vi "Test Bench v18 - TDMS.vi"(5 "Folder to save file to":path=path "C:/Users/LAV-UFSC-2023/Documents/LAV-TCC/Dados-Experimentos/Dados-Bancada-LABVIEW", 6 "Signal Output\nControl":enum32{"White Noise", "Harmonic"}(tab), 7 "stop":bool, 8 "Enable Display":bool=TRUE, 9 "Accel. 2":bool, 10 "Output":bool=TRUE) -> (0 "New file path":path, 2 "Accel. 1 Raw":dbl[](graph), 3 "Output Signal":dynamicdata(graph))   [LabVIEW 2022 SP3]
uses:
  WhiteNoise.ctl
  <vilib>/Utility/error.llb/DialogType.ctl
  <vilib>/Platform/TimedLoop/XDataNode/timing_clust.ctl
  <vilib>/Platform/TimedLoop/XDataNode/nitl_modes.ctl
  <vilib>/Platform/TimedLoop/XDataNode/wakeup.ctl
  <vilib>/DAQmx/write.llb/DAQmx Write (Analog 2D DBL NChan NSamp).vi
  <vilib>/DAQmx/read.llb/DAQmx Read (Analog 1D DBL 1Chan NSamp).vi
  <vilib>/DAQmx/create/channels.llb/DAQmx Create Channel (AI-Acceleration-Accelerometer).vi
  <vilib>/DAQmx/create/channels.llb/DAQmx Create Channel (AO-Voltage-Basic).vi
  <vilib>/DAQmx/configure/timing.llb/DAQmx Timing (Sample Clock).vi
  <vilib>/DAQmx/miscellaneous.llb/DAQmx Fill In Error Info.vi
  <vilib>/platform/TimedLoop/XDataNode/XDataNode.xnode
  <vilib>/measure/NI_MABase.lvlib
  <vilib>/Platform/TimedLoop/XDataNode/XDNodeRunTimeDep.lvlib
  <resource>/objmgr/daqmx.rc
panel:
  in  "Sample Rate":dbl=41200.0
  in  "samples per channel":i32=41200
  out "Frame 2 Duration":i64
  out "Frame 1 Duration":i64
  in  "White Noise\nParameters":T2={"Seed"=0.0, "Standard Deviation"=2.0, "Reset"=FALSE, "Iterator"=1.0, "Seed"=-1, "Lower Cut-Off"=5.0, "Upper Cut-Off"=350.0} {"Upper Cut-Off" min=5.0 max=350.0 step=10.0; "Lower Cut-Off" min=5.0 max=350.0 step=10.0; "Standard Deviation" min=0.001 max=3.0 step=0.05 format="%0.2p"}
  in  "Hamonic\nParameters":T3={"Waveform Type"=0, "Frequency"=10.0, "Amplitude"=0.25} {"Frequency" min=5.0 max=350.0 step=10.0 format="%0.2p"; "Waveform Type" items=["Sine Wave", "Triangle Wave", "Square Wave", "Sawtooth Wave"]; "Amplitude" min=0.001 max=0.3 step=0.05 format="%0.2p"}
  # "Filter"
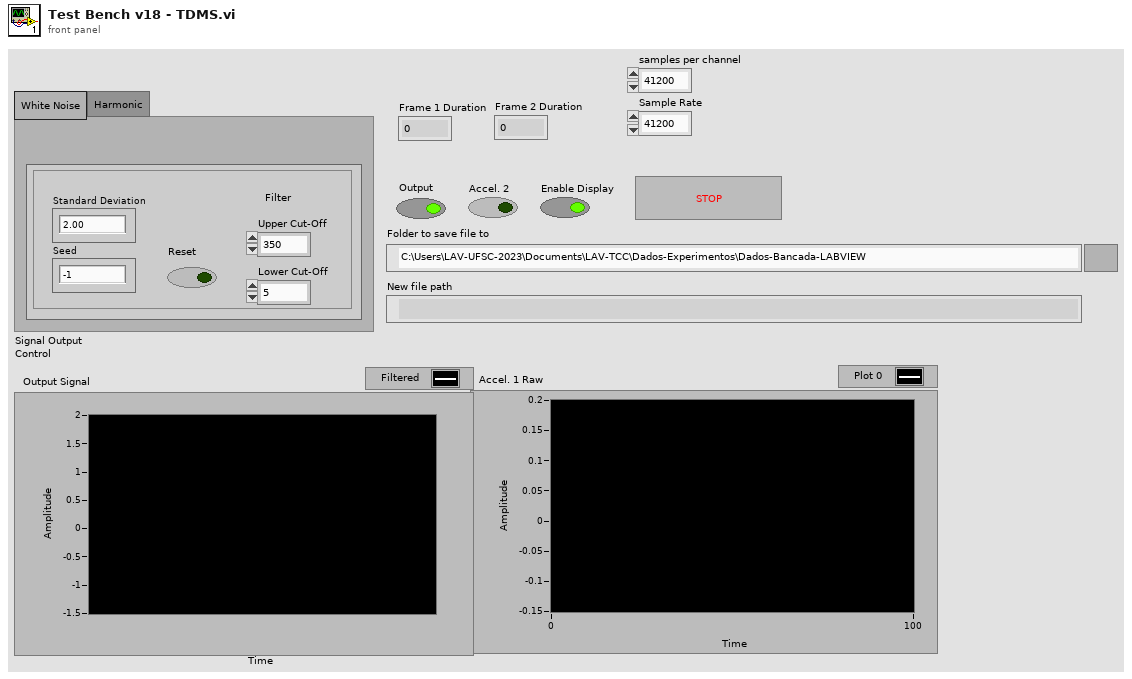
[diagram p1: front panel]
types:
  T1 = typedef "WhiteNoise.ctl" = dbl
  T2 = cluster{"Seed":T1, "Standard Deviation":dbl, "Reset":bool, "Iterator":dbl, "Seed":i8, "Lower Cut-Off":dbl, "Upper Cut-Off":dbl}
  T3 = cluster{"Waveform Type":u16, "Frequency":dbl, "Amplitude":dbl}
  T4 = typedef "DialogType.ctl" = u16
  T5 = enum16{"open", "open or create", "create or replace", "create", "open (read-only)"}
  T6 = typedef "XDNodeRunTimeDep.lvlib/timing_clust.ctl" = cluster{"Expected End [f-1]":u64, "Actual End [f-1]":u64, "Finished Late? [f-1]":bool, "Expected End [i-1]":u64, "Actual End [i-1]":u64, "Finished Late? [i-1]":bool, "Expected Start [i]":u64, "Actual Start [i]":u64, "Expected Start [f]":u64, "Actual Start [f]":u64, "Source Name":string, "Structure Name":string, "Period":i64, "Deadline":i64, "Offset":i64, "Start":i64, "Priority":i32, "Timeout":i32, "Mode":T7, "Wakeup Reason":T8, "Error":errorcluster, "Source Type":string, "Secondary Source Type":string, "Global End Time":u64, "Global Start Time":u64, "Frame Duration":u64, "Iteration Duration":u64, "Assigned CPU":i32, "I/O Scan Engine Mode":u32}
  T7 = typedef "XDNodeRunTimeDep.lvlib/nitl_modes.ctl" = enum32{"No Change", "Process missed periods, maintain original phase", "Discard missed periods, maintain original phase", "Process missed periods, ignore original phase", "Discard missed periods, ignore original phase"}
  T8 = typedef "XDNodeRunTimeDep.lvlib/wakeup.ctl" = enum32{"Normal", "Aborted", "Asynchronous wakeup", "Timing source error", "Timed loop error", "Timeout"}
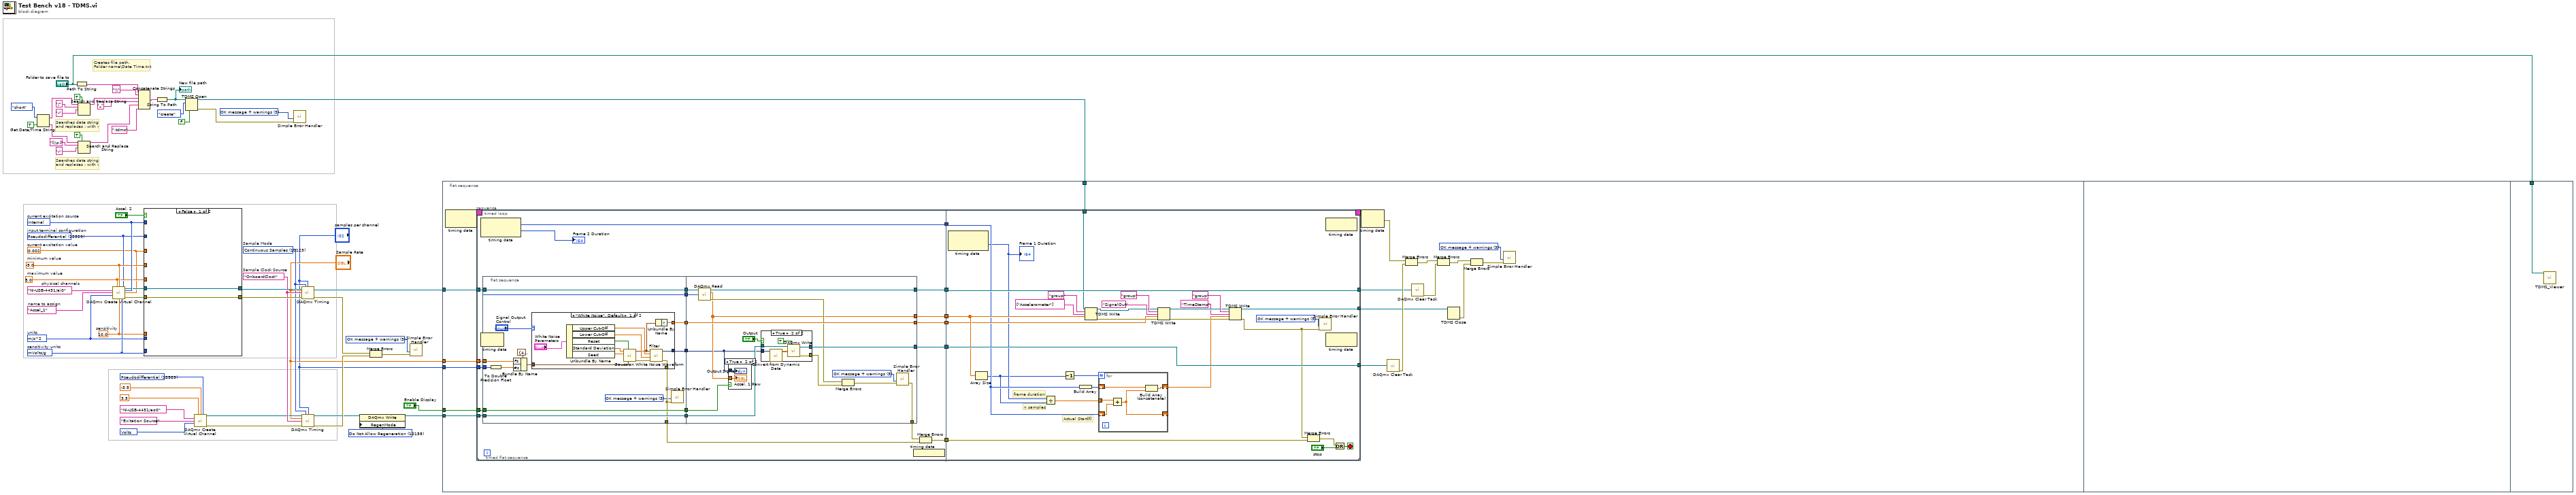
[diagram p0: block diagram]
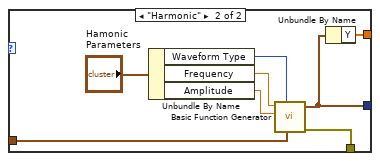
[diagram p2: hidden frame]
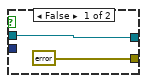
[diagram p4: hidden frame]
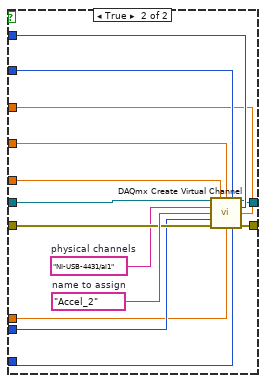
[diagram p5: hidden frame]
diagram:
  w1 = 10158 items=["Allow Regeneration"=10097, "Do Not Allow Regeneration"=10158] ("RegenMode")
  w13 = T4 3 items=["no dialog", "OK message", "continue or stop message", "OK message + warnings", "continue/stop + warnings"] ("type of dialog (OK msg:1)")
  w15 = T4 3 items=["no dialog", "OK message", "continue or stop message", "OK message + warnings", "continue/stop + warnings"] ("type of dialog (OK msg:1)")
  w47 = 12529 items=["Default"=-1, "RSE"=10083, "Differential"=10106, "Pseudodifferential"=12529] ("output terminal configuration")
  w45 = 10348 items=["Volts"=10348, "From Custom Scale"=10065] ("units")
  w51 = 12509 items=["mVolts/g"=12509, "Volts/g"=12510]  # sensitivity units
  w42 = 10.0  # sensitivity
  w50 = 0.002  # current excitation value
  w58 = 10200 items=["Internal"=10200, "External"=10167, "None"=10230]  # current excitation source
  w52 = tag "NI-USB-4431/ai0"  # physical channels
  w39 = tag "OnboardClock"  # Sample Clock Source
  w38 = 10123 items=["Finite Samples"=10178, "Continuous Samples"=10123, "Hardware Timed Single Point"=12522]  # Sample Mode
  w54 = 12529 items=["default"=-1, "RSE"=10083, "NRSE"=10078, "Differential"=10106, "Pseudodifferential"=12529]  # input terminal configuration
  w57 = -5.0  # minimum value
  w56 = 5.0  # maximum value
  w60 = "Accel_1"  # name to assign
  w55 = 12470 items=["g"=10186, "m/s^2"=12470, "in/s^2"=12471, "From Custom Scale"=10065]  # units
  # "Searches date string\nand replaces : with -"
  # "Searches date string\nand replaces : with -"
  # "Creates file path.\nFolder name\\Date Time.txt"
  n1 = Get Date/Time String(date format (0)=enum16{"short", "long", "abbreviated"}."short", want seconds? (F)=TRUE) -> (date string=w18:string, time string=w31:string)  [unwired: 1 in]
  n2 = Path To String(path="Folder to save file to") -> (string=w26:string)
  n3 = Search and Replace String(replace all?=TRUE ("replace all? (F)"), input string=w18, search string="/" ("replace string (\"\")"), replace string="-" ("replace string (\"\")")) -> (result string=w17:string)  [unwired: 4 in, 3 out]
  n4 = Search and Replace String(replace all?=TRUE ("replace all? (F)"), input string=w31, search string="[\\s:]" ("replace string (\"\")"), replace string="-" ("replace string (\"\")")) -> (result string=w24:string)  [unwired: 4 in, 3 out]
  n5 = call-poly <vilib>:"DAQmx Create Virtual Channel.vi"("maximum value"=w56, "minimum value"=w57, "input terminal configuration"=w54, "physical channels"=w52, "current excitation source"=w58, "name to assign"=w60, "current excitation value"=w50, "units"=w55, "sensitivity"=w42, "sensitivity units"=w51) -> ("task out"=w53:refnum<k21>, "error out"=w59:errorcluster)  [unwired: 4 in]
  n6 = Concatenate Strings(w26, "\\" ("string"), w17, "_" ("string"), w24, ".tdms" ("string")) -> (w22:string)
  n7 = case shown="False" "Accel. 2" {
    tunnel: w59 -> [w62 w75]
    tunnel: w58 -> [_ w74]
    tunnel: w57 -> [_ w73]
    tunnel: w56 -> [_ w72]
    tunnel: w55 -> [_ w71]
    tunnel: w54 -> [_ w70]
    tunnel: w53 -> [w61 w69]
    tunnel: w51 -> [_ w67]
    tunnel: w50 -> [_ w66]
    tunnel: w42 -> [_ w65]
    tunnel: [w62 w64] -> w41
    tunnel: [w61 w63] -> w40
    frame False {
    }
    frame True {
      w68 = tag "NI-USB-4431/ai1"  # physical channels
      w76 = "Accel_2"  # name to assign
      n8 = call-poly <vilib>:"DAQmx Create Virtual Channel.vi"("task in"=w69, "maximum value"=w72, "minimum value"=w73, "input terminal configuration"=w70, "physical channels"=w68, "current excitation source"=w74, "name to assign"=w76, "current excitation value"=w66, "units"=w71, "error in"=w75, "sensitivity"=w65, "sensitivity units"=w67) -> ("task out"=w63:refnum<k21>, "error out"=w64:errorcluster)  [unwired: 2 in]
    }
  }
  n9 = String To Path(string=w22) -> (path=w8:path)
  "New file path" <- w8
  n10 = TDMS Open(6:FALSE ("enable asynchronous? (T)"), 10:T5."create" ("operation (0:open)"), 11:w8) -> (0:w4:errorcluster, 3:w5:refnum<k34>)  [unwired: 4 in]
  n11 = call-poly <vilib>:"DAQmx Create Virtual Channel.vi"("maximum value"=3.5, "minimum value"=-3.5, "output terminal configuration"=w47, "physical channels"=tag "NI-USB-4431/ao0", "name to assign"="Exitation Source", "units"=w45) -> ("task out"=w36:refnum<k21>, "error out"=w37:errorcluster)  [unwired: 8 in]
  n12 = call <vilib>:"Simple Error Handler.vi"("type of dialog (OK msg:1)"=w15, "error in (no error)"=w4) -> ()  [unwired: 3 in, 5 out]
  n13 = call-poly <vilib>:"DAQmx Timing.vi"("task/channels in"=w40, "sample mode"=w38, "samples per channel"="samples per channel", "rate"="Sample Rate", "source"=w39, "error in"=w41) -> ("task out"=w12:refnum<k21>, "error out"=w44:errorcluster)  [unwired: 8 in]
  n14 = call-poly <vilib>:"DAQmx Timing.vi"("task/channels in"=w36, "sample mode"=w38, "samples per channel"="samples per channel", "rate"="Sample Rate", "source"=w39, "error in"=w37) -> ("task out"=w3:refnum<k21>, "error out"=w35:errorcluster)  [unwired: 8 in]
  n15 = property class="DAQmx Write"(reference=w3, "RegenMode"=w1) -> (reference out=w2:refnum<k21>)  [unwired: 1 in, 1 out]
  n16 = Merge Errors(w44, w35) -> (w11:errorcluster)
  n17 = call <vilib>:"Simple Error Handler.vi"("type of dialog (OK msg:1)"=w13, "error in (no error)"=w11) -> ()  [unwired: 3 in, 5 out]
  n18 = flat-sequence {
    tunnel: w2 -> [w92]
    tunnel: w12 -> [w90]
    tunnel: w5 -> [w82]
    tunnel: "Enable Display" -> [w89]
    tunnel: "Sample Rate" -> [w81]
    tunnel: "samples per channel" -> [w80]
    tunnel: "Folder to save file to" -> [w243]
    frame #0 {
      w93 = T4 3 items=["no dialog", "OK message", "continue or stop message", "OK message + warnings", "continue/stop + warnings"] ("type of dialog (OK msg:1)")
      n19 = node-c288() -> (w95:T6)  [unwired: 1 in]
      n20 = timed-loop {
        tunnel: w92 -> [w104]
        tunnel: [w103] -> w91
        tunnel: w90 -> [w102]
        tunnel: [w98] -> w87
        tunnel: [w96] -> w79
        tunnel: w89 -> [w101]
        tunnel: w80 -> [w100]
        timing: w95 -> [_]
        timing-out: [_] -> w94
        tunnel: w82 -> [w99]
        tunnel: w81 -> [w97]
        stop <- w225 stop-if-true
        n21 = timed-sequence {
          timing: _ -> [_]
          timing-out: _ -> [_]
          tunnel: w104 -> [w119]
          tunnel: [w118] -> w103
          tunnel: w102 -> [w117]
          tunnel: w101 -> [w116]
          tunnel: w100 -> [w115]
          tunnel: w99 -> [w111]
          tunnel: [w110] -> w98
          tunnel: w97 -> [w107]
          tunnel: [w106] -> w96
          n22 = timed-flat-sequence {
            tunnel: w119 -> [w133]
            tunnel: w117 -> [w132]
            tunnel: w116 -> [w129]
            tunnel: w115 -> [w128]
            tunnel: [w131] -> w114
            tunnel: [w130] -> w113
            tunnel: [w125] -> w112
            tunnel: [w124] -> w109
            tunnel: [w123] -> w108
            tunnel: w107 -> [w122]
            tunnel: [w121] -> w105
            tunnel: [w229] -> w118
            tunnel: w114 -> [w229]
            tunnel: w113 -> [w223]
            tunnel: w112 -> [w226]
            tunnel: w111 -> [w212]
            tunnel: [w223] -> w110
            tunnel: w109 -> [w221]
            tunnel: w108 -> [w213]
            tunnel: [w217] -> w106
            tunnel: w105 -> [w206]
            frame #0 {
              n23 = node-c288() -> (w121:i64, →"Frame 2 Duration":i64)  [unwired: 1 in]
              n24 = flat-sequence {
                tunnel: [w153] -> w139
                tunnel: [w149] -> w138
                tunnel: [w152] -> w137
                tunnel: [w150] -> w136
                tunnel: [w151] -> w135
                tunnel: [w145] -> w134
                tunnel: [w148] -> w126
                tunnel: w133 -> [w152]
                tunnel: w132 -> [w153]
                tunnel: w129 -> [w150]
                tunnel: w128 -> [w145]
                tunnel: w122 -> [w146]
                tunnel: w139 -> [w183]
                tunnel: w138 -> [w190]
                tunnel: w137 -> [w188]
                tunnel: w136 -> [w184]
                tunnel: w135 -> [w177]
                tunnel: w134 -> [w182]
                tunnel: [w178] -> w127
                tunnel: [w181] -> w124
                tunnel: [w190] -> w123
                tunnel: [w187] -> w131
                tunnel: [w185] -> w130
                frame #0 {
                  w147 = T4 3 items=["no dialog", "OK message", "continue or stop message", "OK message + warnings", "continue/stop + warnings"] ("type of dialog (OK msg:1)")
                  n25 = To Double Precision Float(number=w145) -> (double precision float=w144:dbl)
                  n26 = Bundle By Name(cluster=cluster{"Fs":dbl, "#s":dbl} {"Fs"=41200.0, "#s"=41200.0} ("sampling info"), "Fs"=w146, "#s"=w144) -> (w155:cluster{"Fs":dbl, "#s":dbl})
                  n27 = case shown="\"White Noise\", Default" "Signal Output\nControl" {
                    tunnel: w155 -> [w166 w175]
                    tunnel: [w159 w171] -> w151
                    tunnel: [w158 w170] -> w149
                    tunnel: [w157 w169] -> w148
                    frame "White Noise", Default {
                      n28 = Unbundle By Name("White Noise\nParameters") -> ("Upper Cut-Off"=w162:dbl, "Lower Cut-Off"=w161:dbl, "Reset"=w163:bool, "Standard Deviation"=w164:dbl, "Seed"=w165:T1)
                      n29 = call <vilib>:"Gaussian White Noise Waveform.vi"("sampling info"=w166, "reset signal"=w163, "seed"=w165, "standard deviation"=w164) -> ("error out"=w168:errorcluster, "signal out"=w160:waveform(dbl))  [unwired: 6 in]
                      n30 = call "Filter"("error in (no error)"=w168, "Lower Cut-Off"=w161, "Upper Cut-Off"=w162, "Signal"=w160) -> ("error out"=w157:errorcluster, "Filtered Signal"=w159:dynamicdata)  [unwired: 6 in]
                      n31 = Unbundle By Name(w160) -> ("Y"=w158:dbl[])
                    }
                    frame "Harmonic" {
                      n32 = Unbundle By Name("Hamonic\nParameters") -> ("Waveform Type"=w174:u16, "Frequency"=w173:dbl, "Amplitude"=w172:dbl)
                      n33 = call <vilib>:"Basic Function Generator.vi"("sampling info"=w175, "signal type"=w174, "amplitude"=w172, "frequency"=w173) -> ("error out"=w169:errorcluster, "signal out"=w171:waveform(dbl))  [unwired: 5 in, 1 out]
                      n34 = Unbundle By Name(w171) -> ("Y"=w170:dbl[])
                    }
                  }
                  n35 = call <vilib>:"Simple Error Handler.vi"("type of dialog (OK msg:1)"=w147, "error in (no error)"=w148) -> ()  [unwired: 3 in, 5 out]
                }
                frame #1 {
                  w180 = T4 3 items=["no dialog", "OK message", "continue or stop message", "OK message + warnings", "continue/stop + warnings"] ("type of dialog (OK msg:1)")
                  n36 = call-poly <vilib>:"DAQmx Read.vi"("task/channels in"=w183, "number of samples per channel"=w182) -> ("task out"=w185:refnum<k21>, "data"=w181:dbl[], "error out"=w186:errorcluster)  [unwired: 11 in]
                  n37 = case shown="True" w184 {
                    tunnel: w181 -> [_ w192]
                    tunnel: w177 -> [_ w191]
                    frame False {
                    }
                    frame True {
                      "Accel. 1 Raw" <- w192
                      "Output Signal" <- w191
                    }
                  }
                  n38 = case shown="True" "Output" {
                    tunnel: w188 -> [w194 w200]
                    tunnel: [errorcluster {"status"=FALSE, "code"=0, "source"=""} ("error out") w198] -> w179
                    tunnel: [w194 w199] -> w187
                    tunnel: w177 -> [_ w197]
                    frame False {
                    }
                    frame True {
                      n39 = call "Convert from Dynamic Data"("Dynamic Data Type"=w197) -> ("Array"=w196:dbl[][])  [unwired: 3 in]
                      n40 = call-poly <vilib>:"DAQmx Write.vi"("task/channels in"=w200, "auto start"=TRUE, "data"=w196) -> ("task out"=w199:refnum<k21>, "error out"=w198:errorcluster)  [unwired: 10 in, 1 out]
                    }
                  }
                  n41 = Merge Errors(w186, w179) -> (w178:errorcluster)
                  n42 = call <vilib>:"Simple Error Handler.vi"("type of dialog (OK msg:1)"=w180, "error in (no error)"=w178) -> ()  [unwired: 3 in, 5 out]
                }
              }
              n43 = node-c288() -> ()  [unwired: 1 out]
              n44 = Merge Errors(w127, w126) -> (w125:errorcluster)
            }
            frame #1 {
              w224 = T4 3 items=["no dialog", "OK message", "continue or stop message", "OK message + warnings", "continue/stop + warnings"] ("type of dialog (OK msg:1)")
              # "Actual Start[f]"
              # "n samples"
              # "frame duration"
              n45 = node-c288() -> (w205:i64)  [unwired: 1 in, 1 out]
              "Frame 1 Duration" <- w205
              n46 = Array Size(array=w221) -> (size(s)=w204:i32)
              n47 = Divide(x=w205, y=w204) -> (x/y=w201:dbl)
              n48 = Decrement(x=w204) -> (x-1=w203:i32)
              n49 = Build Array(w206) -> (w202:i64[])
              n50 = TDMS Write(0:w212, 5:"group" ("group name in (Untitled)"), 7:string[] ["Accelerometer"] ("channel name(s) in (Untitled)"), 9:w221) -> (4:w211:refnum<k34>, 15:w215:errorcluster)  [unwired: 2 in, 2 out]
              n51 = for {
                N: w203 -> [_]
                shift-right: [w230] -> _
                shift-left: w206 -> [w234]
                tunnel: w201 -> [w233]
                shift-right: [w232] -> w207
                shift-left: w202 -> [w231]
                n52 = Add(x=w233, y=w234) -> (x+y=w230:dbl)
                n53 = Build Array (concatenate)(w231, w230) -> (w232:dbl[])
              }
              n54 = TDMS Write(0:w211, 5:"group" ("group name in (Untitled)"), 7:"SignalOut", 9:w213, 11:w215) -> (4:w210:refnum<k34>, 15:w214:errorcluster)  [unwired: 1 in, 2 out]
              n55 = TDMS Write(0:w210, 5:"group" ("group name in (Untitled)"), 7:"TimeStamp", 9:w207, 11:w214) -> (4:w217:refnum<k34>, 15:w209:errorcluster)  [unwired: 1 in, 2 out]
              n56 = Merge Errors(w209, w226) -> (w228:errorcluster)
              n57 = call <vilib>:"Simple Error Handler.vi"("type of dialog (OK msg:1)"=w224, "error in (no error)"=w209) -> ()  [unwired: 3 in, 5 out]
              n58 = node-c288() -> ()  [unwired: 1 in, 1 out]
              n59 = Or(x=w228, y="stop") -> (x .or. y?=w225:bool)
            }
          }
        }
        n60 = node-c288() -> ()  [unwired: 1 in, 1 out]
        n61 = node-c288() -> ()  [unwired: 1 in, 1 out]
      }
      n62 = node-c288(w94) -> (w83:errorcluster)
      n63 = call <vilib>:"DAQmx Clear Task.vi"("task in"=w91) -> ("error out"=w88:errorcluster)  [unwired: 14 in]
      n64 = Merge Errors(w83, w88) -> (w86:errorcluster)
      n65 = call <vilib>:"DAQmx Clear Task.vi"("task in"=w87) -> ("error out"=w85:errorcluster)  [unwired: 14 in]
      n66 = Merge Errors(w86, w85) -> (w78:errorcluster)
      n67 = TDMS Close(11:w79) -> (0:w77:errorcluster)  [unwired: 1 in, 1 out]
      n68 = Merge Errors(w78, w77) -> (w84:errorcluster)
      n69 = call <vilib>:"Simple Error Handler.vi"("type of dialog (OK msg:1)"=w93, "error in (no error)"=w84) -> ()  [unwired: 3 in, 5 out]
    }
    frame #1 {
    }
    frame #2 {
      n70 = call "TDMS_Viewer.vi"("Data Directory"=w243) -> ()  [unwired: 11 in]
    }
  }
